vi "Need_Interpolation.vi"(1 "Illuminants":string[][](array[string])) -> (0 "Interpolate":bool)   [LabVIEW 2013]
panel:
  out "index":i32
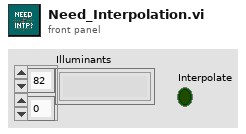
[diagram p1: front panel]
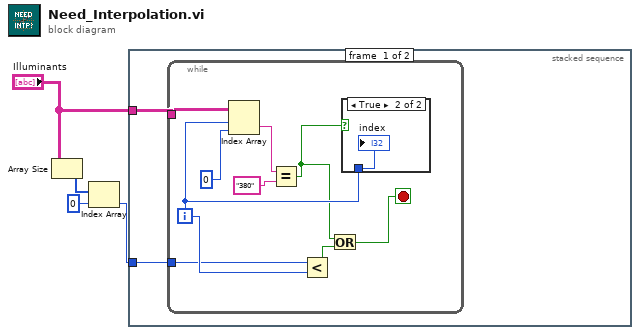
[diagram p0: block diagram]
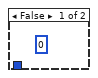
[diagram p2: hidden frame]
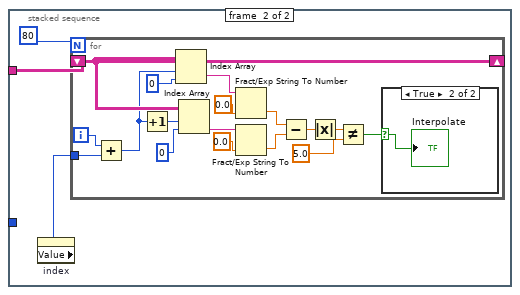
[diagram p3: hidden frame]
diagram:
  n1 = Array Size(array="Illuminants") -> (size(s)=w3:i32[])
  n2 = Index Array(array=w3, index=0) -> (element=w1:i32)
  n3 = stacked-sequence {
    tunnel: "Illuminants" -> [w6 w19]
    tunnel: w1 -> [w5 _]
    frame #0 {
      n4 = while {
        tunnel: w6 -> [w15]
        tunnel: w5 -> [w7]
        i -> [w11]
        stop <- w8 stop-if-true
        n5 = Index Array(array=w15, index (row)=w11, index (col)=0 ("disabled index (col)")) -> (element=w13:string)
        n6 = Equal?(x=w13, y="380") -> (x = y?=w10:bool)
        n7 = Less?(x=w7, y=w11) -> (x < y?=w9:bool)
        n8 = Or(x=w10, y=w9) -> (x .or. y?=w8:bool)
        n9 = case shown="True" w10 {
          tunnel: w11 -> [_ w16]
          frame False {
            (unwired) 0
          }
          frame True {
            "index" <- w16
          }
        }
      }
    }
    frame #1 {
      n10 = property on="index" class="DigNum (strict)"() -> ("Value"=w18:i32)  [unwired: 2 in, 2 out]
      n11 = for {
        N: 80 -> [_]
        shift-right: [w26] -> _
        shift-left: w19 -> [w26]
        tunnel: w18 -> [w20]
        i -> [w21]
        n12 = Add(x=w21, y=w20) -> (x+y=w22:i32)
        n13 = Increment(x=w22) -> (x+1=w24:i32)
        n14 = Index Array(array=w26, index (row)=w22, index (col)=0 ("disabled index (col)")) -> (element=w25:string)
        n15 = Index Array(array=w26, index (row)=w24, index (col)=0 ("disabled index (col)")) -> (element=w27:string)
        n16 = Fract/Exp String To Number(string=w25, default (0 dbl)=0.0 ("default (0 DBL)")) -> (number=w32:dbl)  [unwired: 2 in, 1 out]
        n17 = Fract/Exp String To Number(string=w27, default (0 dbl)=0.0 ("default (0 DBL)")) -> (number=w31:dbl)  [unwired: 2 in, 1 out]
        n18 = Subtract(x=w32, y=w31) -> (x-y=w30:dbl)
        n19 = Absolute Value(x=w30) -> (abs(x)=w29:dbl)
        n20 = Not Equal?(x=w29, y=5.0) -> (x != y?=w23:bool)
        n21 = case shown="True" w23 {
          selector: w23 -> [_ w37]
          frame False {
          }
          frame True {
            "Interpolate" <- w37
          }
        }
      }
    }
  }
